vi "제목없음 2 (SubVI).vi"(1 "A 4":dbl, 2 "A 3":dbl, 3 "A 2":dbl, 4 "A":dbl) -> (0 "x*y":dbl)   [LabVIEW 2017]
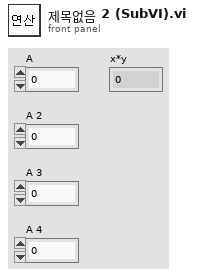
[diagram p1: front panel]
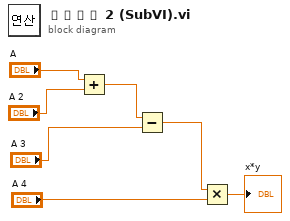
[diagram p0: block diagram]
diagram:
  n1 = Add(x="A", y="A 2") -> (x+y=w3:dbl)
  n2 = Subtract(x=w3, y="A 3") -> (x-y=w5:dbl)
  n3 = Multiply(x=w5, y="A 4") -> (x*y=→"x*y":dbl)
